vi "simple_qa_agent_sm_template.vi"   [LabVIEW 2020]
uses:
  user_interfaces/simple_html_chat_ui/simple_html_chat_ui.lvclass
  models/abstract_llm_base/abstract_llm_base.lvclass
  vectorstore/abstract_vector_base/abstract_vector_base.lvclass
  agent_simple_qa/agent_simple_qa.lvclass
  models/abstract_message_base/abstract_message_base.lvclass
  <vilib>/addons/_JKI Toolkits/State Machine/_JKI_lib_State_Machine.llb/Select State(s)_err__jki_lib_state_machine.vi
  vectorstore/vector_qdrant/vector_qdrant.lvclass
  D:/Personal/LabVIEW LLMs/src/vectorstore/abstract_vector_base/abstract_vector_base.lvclass
  models/llm_openai_chatmodels/llm_openai_chatmodels.lvclass
  D:/Personal/LabVIEW LLMs/src/models/abstract_llm_base/abstract_llm_base.lvclass
  models/llm_openai_embedding/llm_openai_embedding.lvclass
  agent_simple_qa_dynamicdata/agent_simple_qa_dynamic.lvclass
  D:/Personal/LabVIEW LLMs/src/agent/agent_simple_qa/agent_simple_qa.lvclass
  <vilib>/addons/_JKI Toolkits/State Machine/_JKI_lib_State_Machine.llb/Periodic Trigger__ogtk__JKI-SM__jki_lib_state_machine.vi
  models/llm_openai_chatmodels/Instantiate_llm_openai.vi
  models/llm_openai_embedding/Instantiate_llm_openai_embed.vi
  agent_simple_qa/poly/ask_your_model.vi
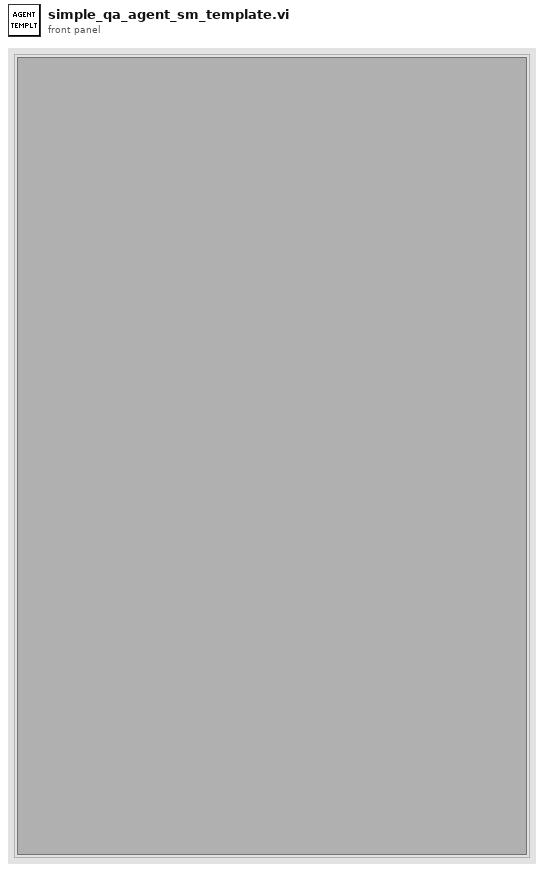
[diagram p1: front panel]
types:
  T1 = enum32{"Invalid", "Standard", "Closed", "Hidden", "Minimized", "Maximized"}
  T2 = enum32{"invalid app kind", "Development System", "Run Time System", "Student Edition", "Embedded LabVIEW", "Evaluation", "Custom"}
  T3 = cluster{"Core":cluster{"Current VI Reference":refnum<vi>, "Close Panel on Exit?":bool}, "Agent":cluster{"UI_Chat":refnum<class "simple_html_chat_ui.lvclass">, "Model_Generative":refnum<class "abstract_llm_base.lvclass">, "Model_Embedding":refnum<class "abstract_llm_base.lvclass">, "Vector Store":refnum<class "abstract_vector_base.lvclass">, "Agent_QA":refnum<class "agent_simple_qa.lvclass">, "last_message":refnum<class "abstract_message_base.lvclass">}}
  T4 = cluster{"UI_Chat":refnum<class "simple_html_chat_ui.lvclass">, "Model_Generative":refnum<class "abstract_llm_base.lvclass">, "Model_Embedding":refnum<class "abstract_llm_base.lvclass">, "Vector Store":refnum<class "abstract_vector_base.lvclass">, "Agent_QA":refnum<class "agent_simple_qa.lvclass">, "last_message":refnum<class "abstract_message_base.lvclass">}
  T5 = cluster{"Current VI Reference":refnum<vi>, "Close Panel on Exit?":bool}
  T6 = typedef "simple_html_chat_ui.lvclass/web_events.ctl" = cluster{"User prompt":refnum<user-event>, "Clear history":refnum<user-event>}
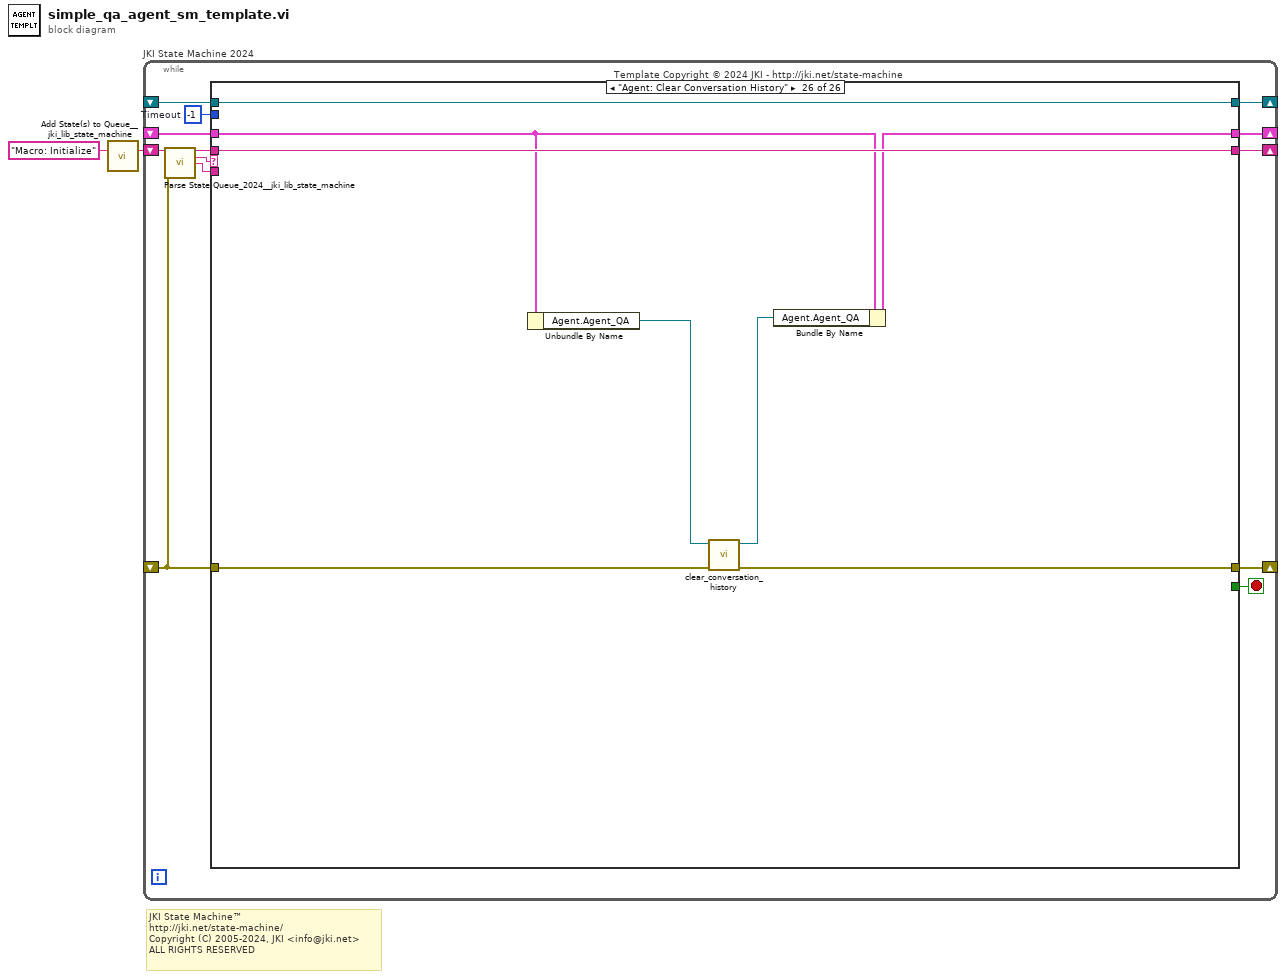
[diagram p0: block diagram]
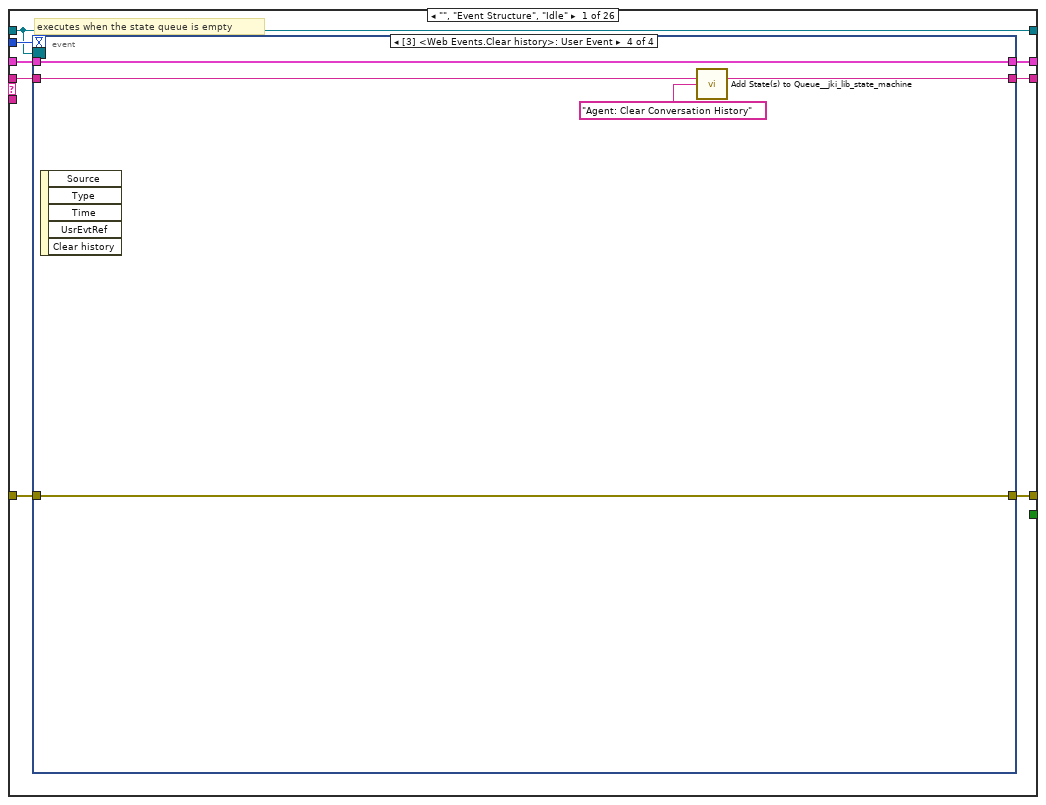
[diagram p2: hidden frame]
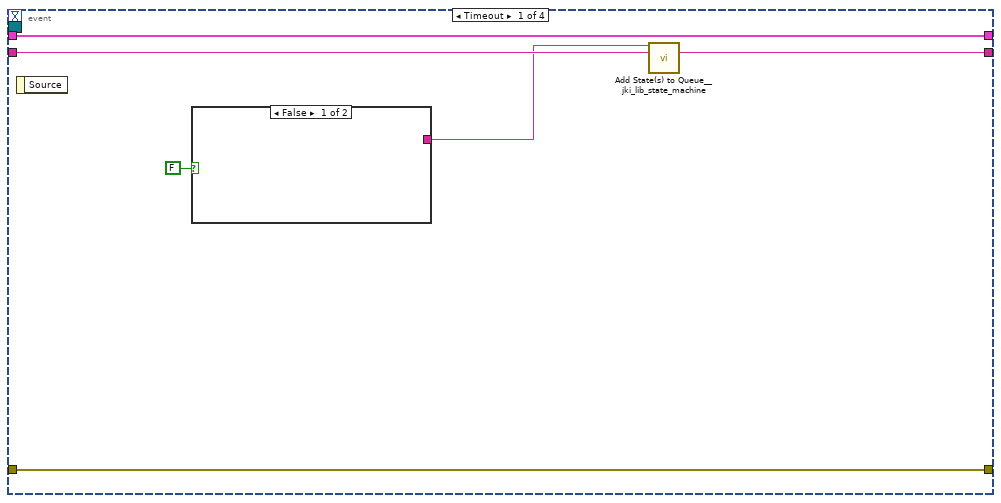
[diagram p3: hidden frame]
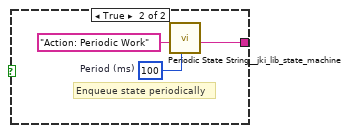
[diagram p4: hidden frame]
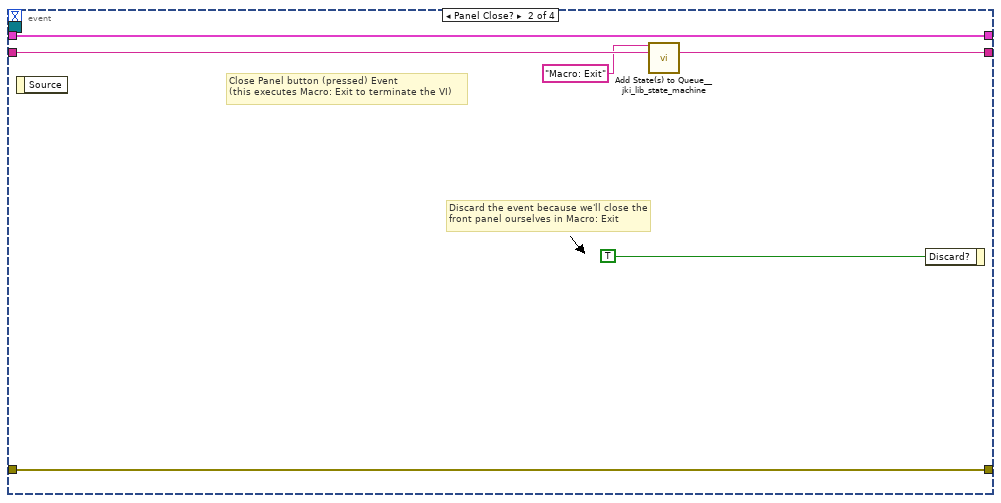
[diagram p5: hidden frame]
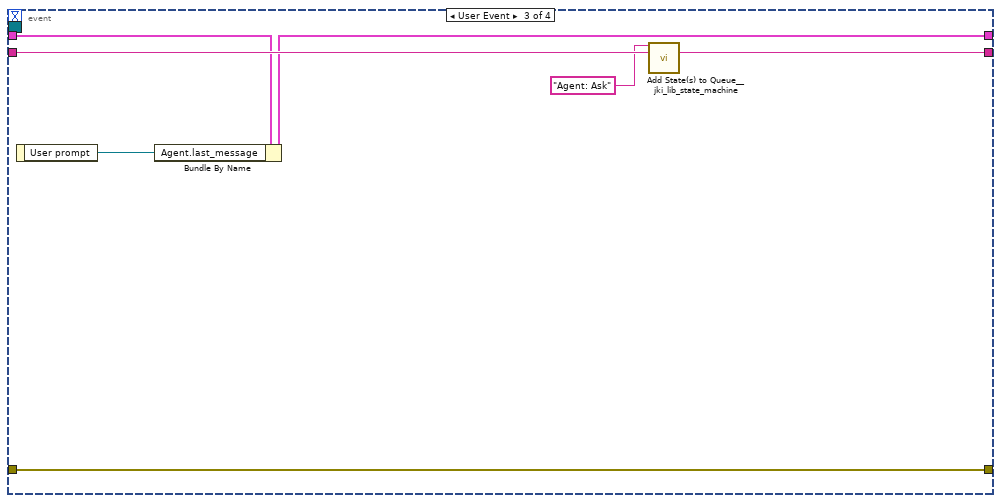
[diagram p6: hidden frame]
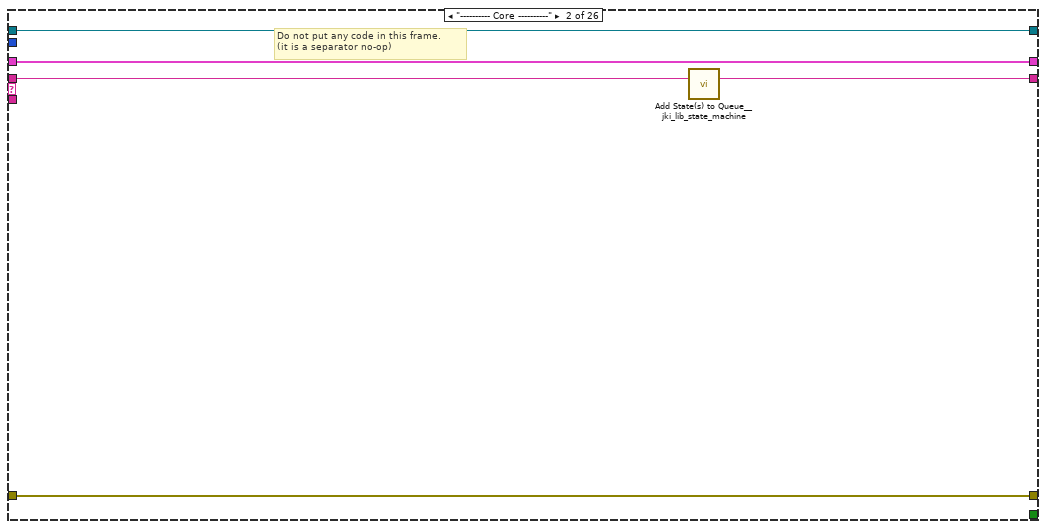
[diagram p7: hidden frame]
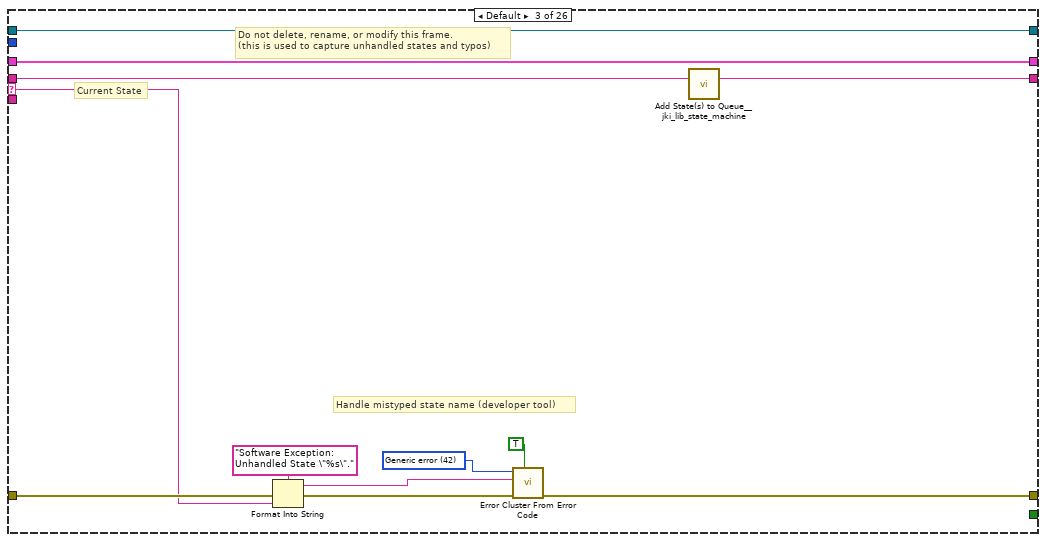
[diagram p8: hidden frame]
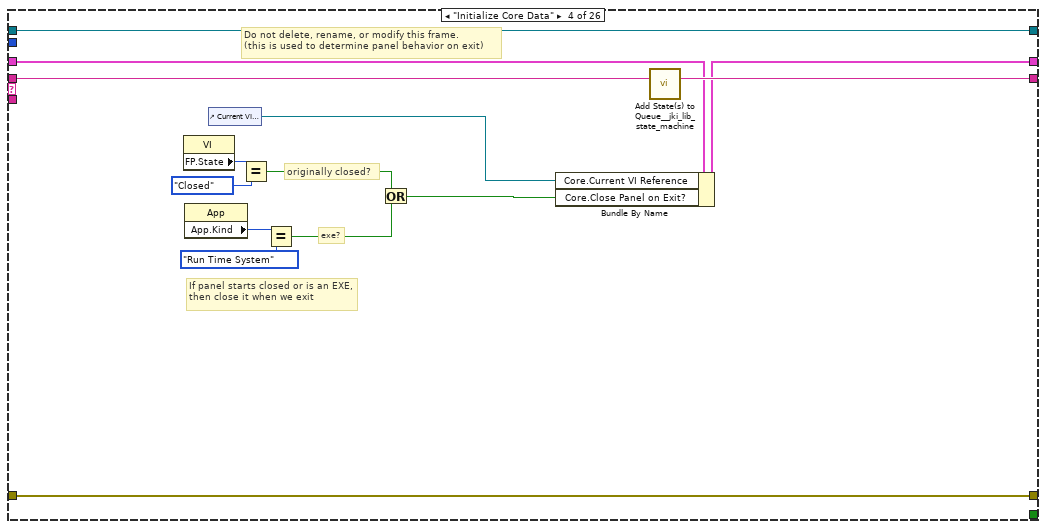
[diagram p9: hidden frame]
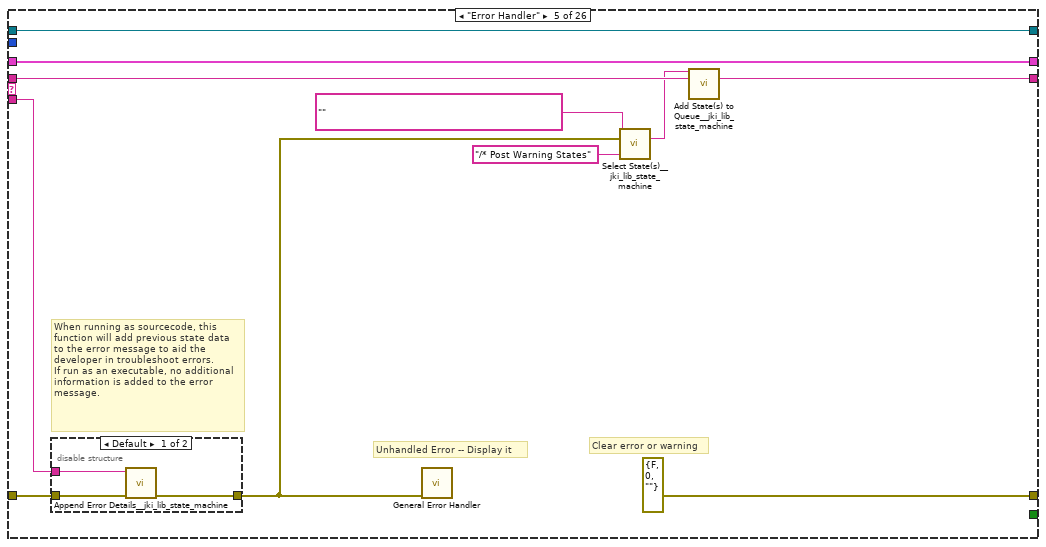
[diagram p10: hidden frame]
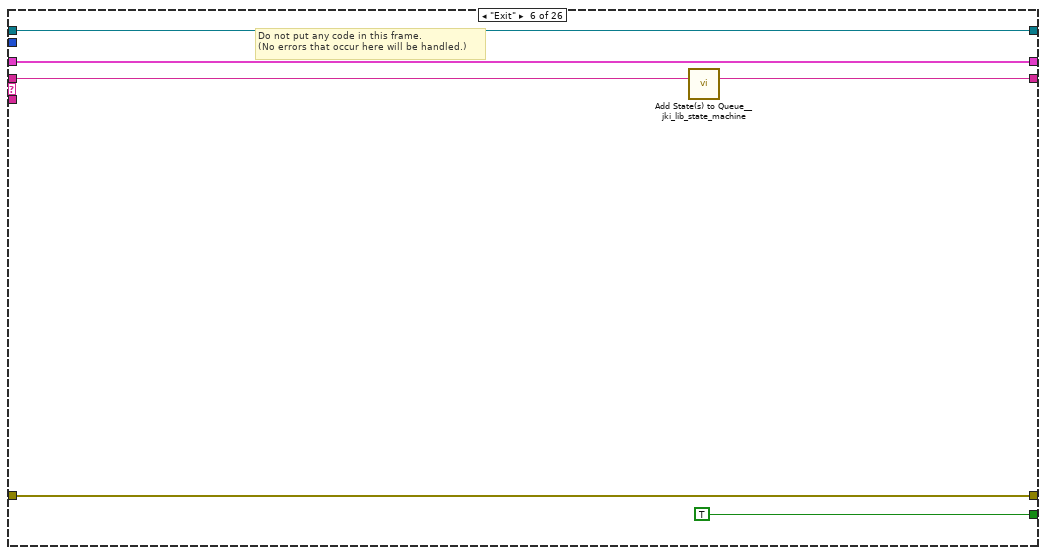
[diagram p12: hidden frame]
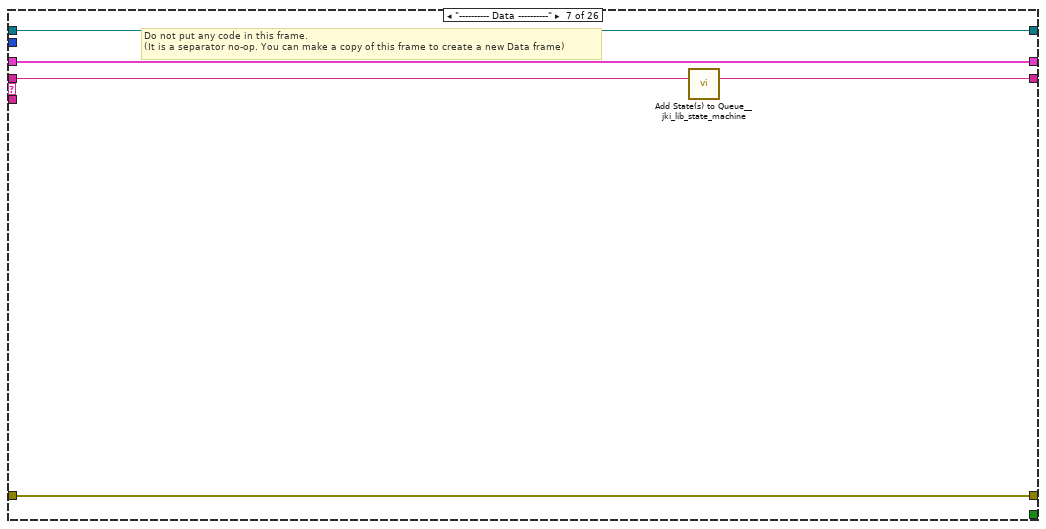
[diagram p13: hidden frame]
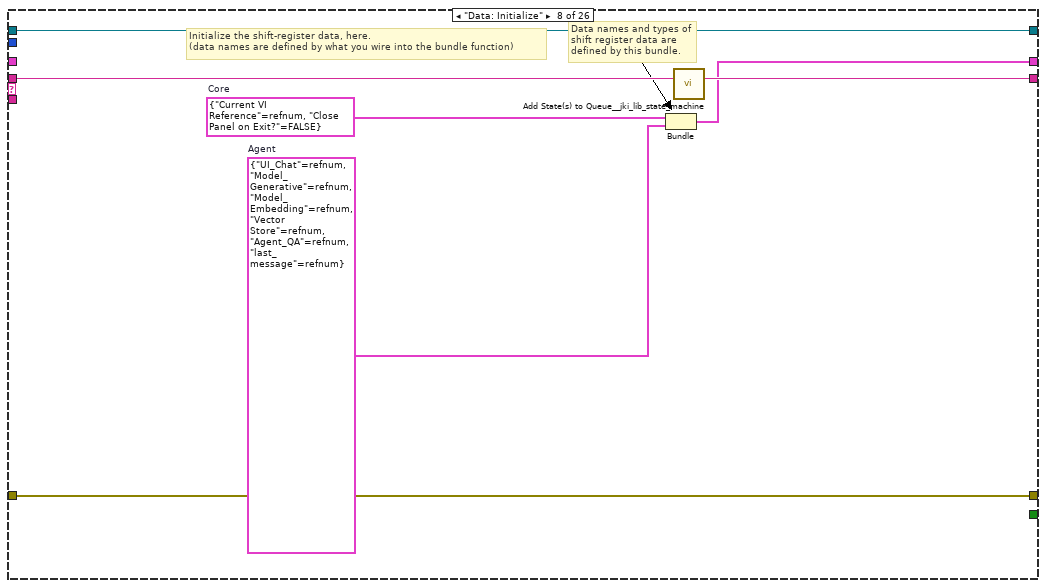
[diagram p14: hidden frame]
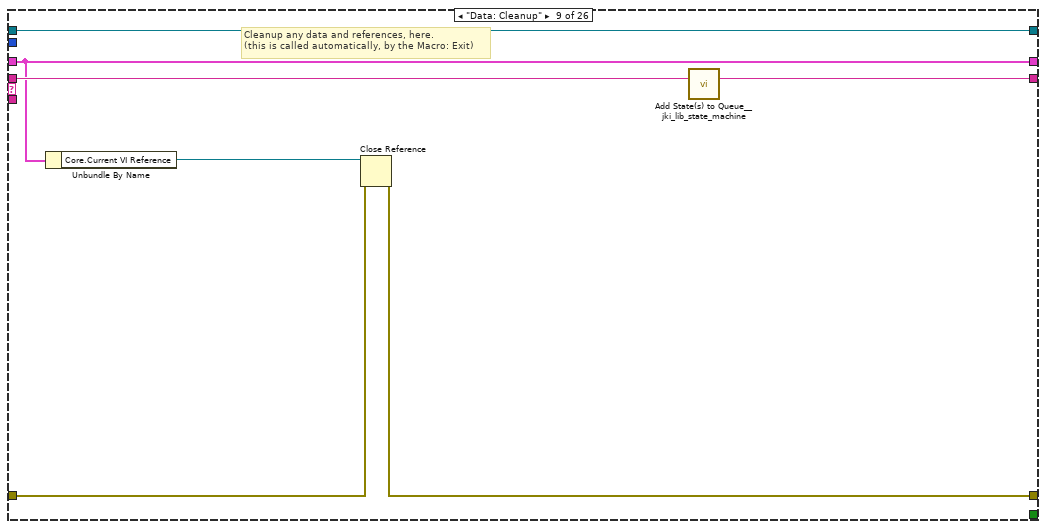
[diagram p15: hidden frame]
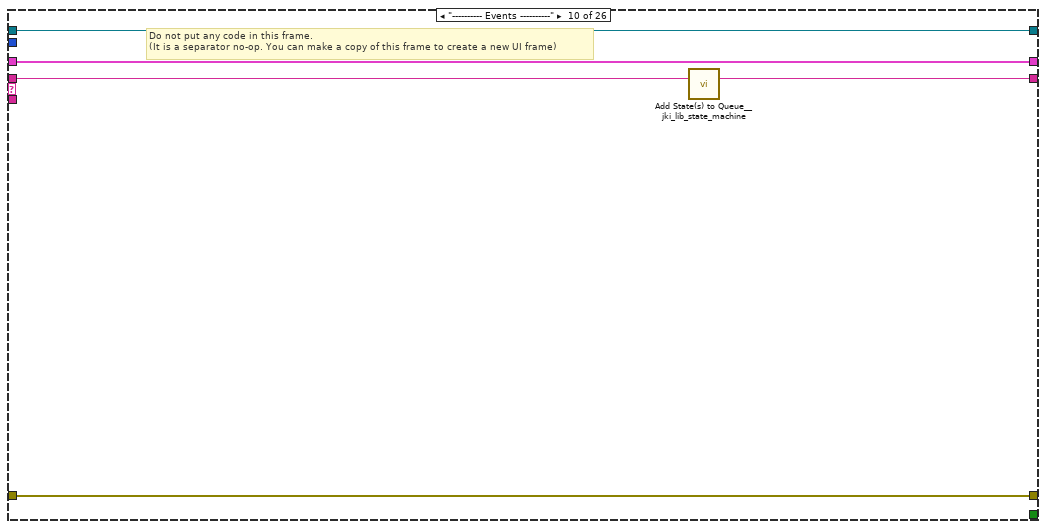
[diagram p16: hidden frame]
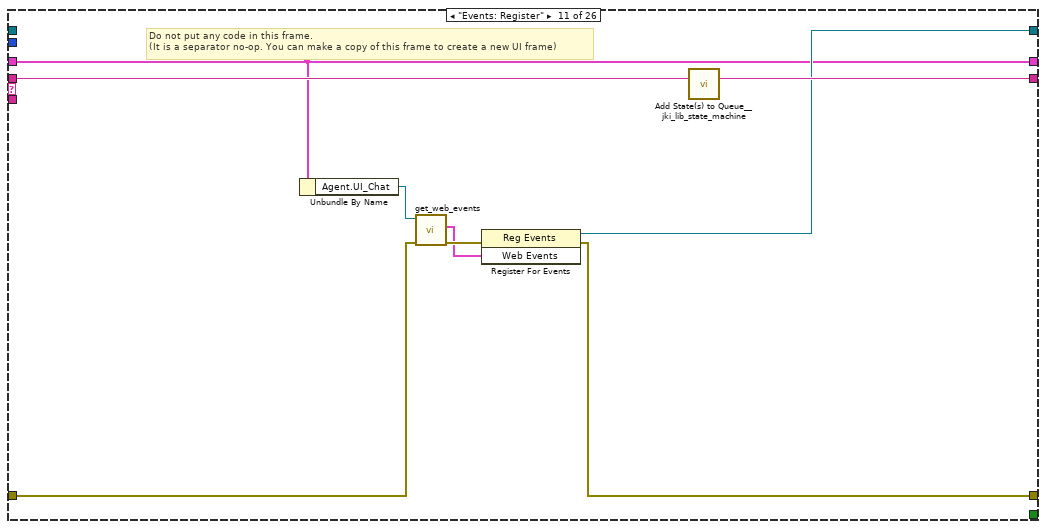
[diagram p17: hidden frame]
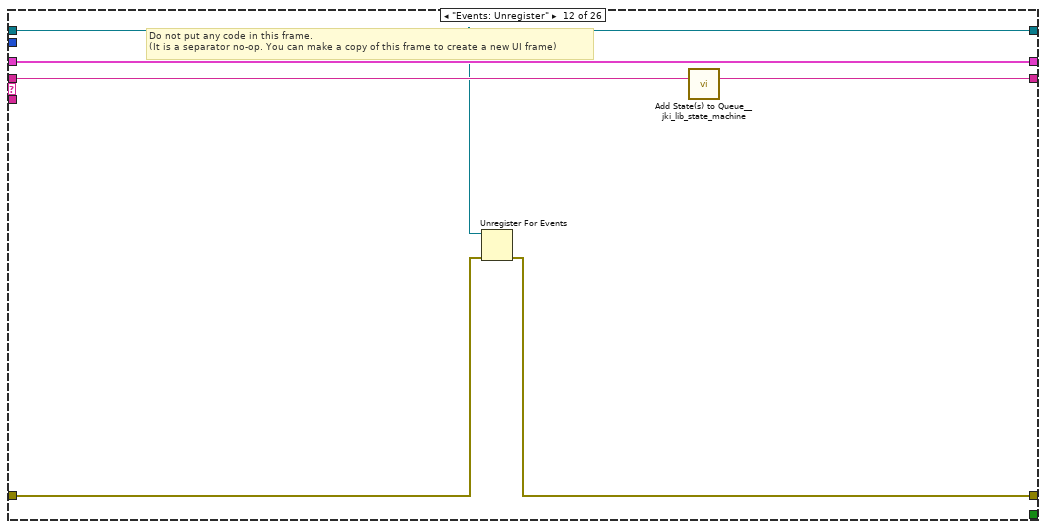
[diagram p18: hidden frame]
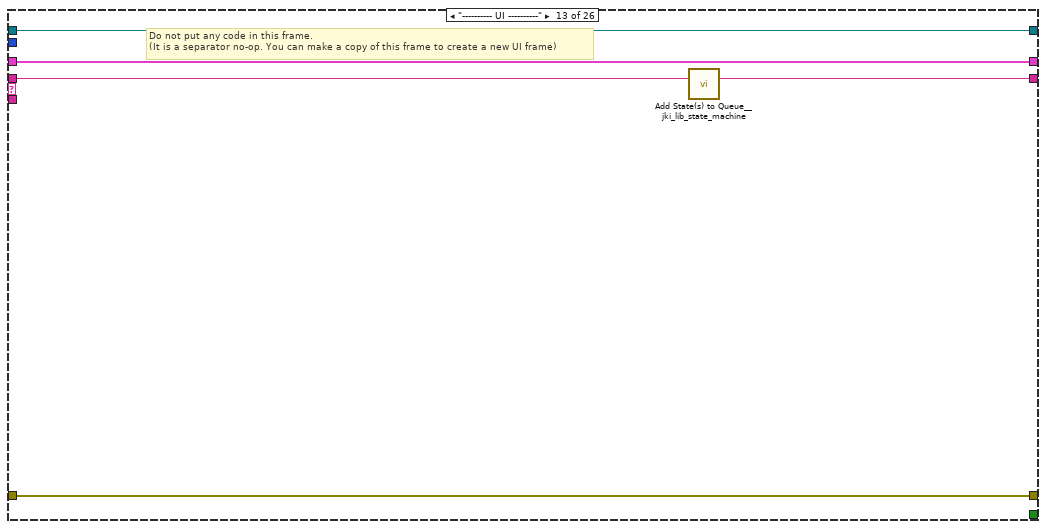
[diagram p19: hidden frame]
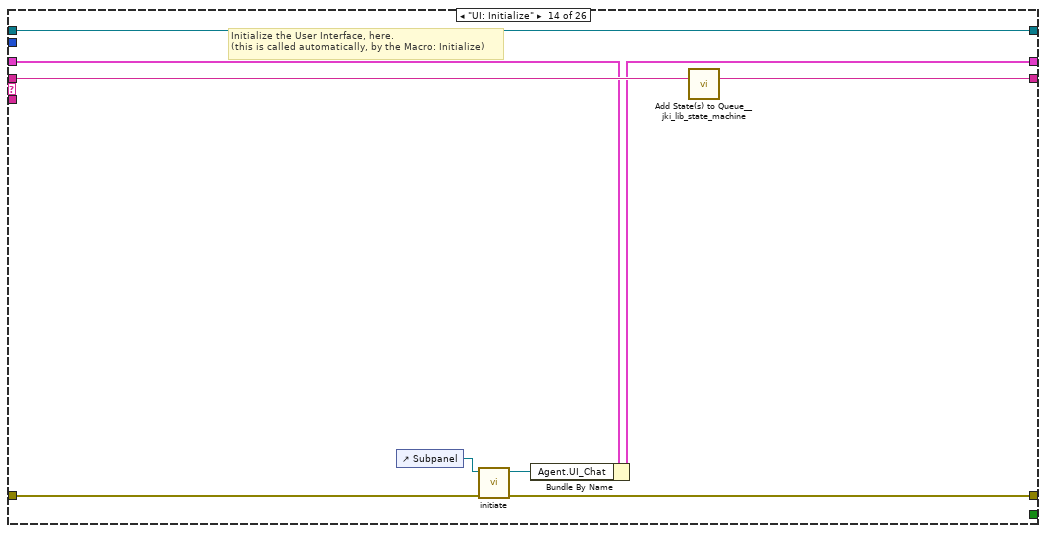
[diagram p20: hidden frame]
diagram:
  # "JKI State Machine™\nhttp://jki.net/state-machine/\nCopyright (C) 2005-2024, JKI <info@jki.net>\nALL RIGHTS RESERVED"
  n1 = call <vilib>:"Add State(s) to Queue__jki_lib_state_machine.vi"("State(s) in (\"\")"="Macro: Initialize") -> ("States Out"=w2:string)  [unwired: 14 in]
  n2 = while "JKI State Machine 2024" {
    shift-right: [w8] -> _
    shift-left: _ -> [w7]
    shift-right: [w11] -> _
    shift-left: _ -> [w5]
    shift-right: [w10] -> _
    shift-left: w2 -> [w12]
    shift-right: [w4] -> _
    shift-left: _ -> [w3]
    stop <- w9 stop-if-true
    w6 = -1  # Timeout
    # "Template Copyright © 2024 JKI - http://jki.net/state-machine"
    n3 = call <vilib>:"Parse State Queue_2024__jki_lib_state_machine.vi"("State Queue"=w12, "Error In (no error)"=w5) -> ("Remaining States"=w14:string, "Current State"=w15:string, "Arguments"=w13:string)  [unwired: 11 in]
    n4 = case shown="\"Agent: Clear Conversation History\"" w15 {
      selector: w15 -> [_ _ w57 _ _ _ _ _ _ _ _ _ _ _ _ _ _ _ _ _ _ _ _ _ _ _]
      tunnel: w14 -> [w23 w55 w61 w81 w92 w102 w107 w114 w121 w126 w135 w141 w146 w155 w162 w172 w179 w191 w261 w267 w277 w282 w307 w320 w332 w339]
      tunnel: w13 -> [_ _ _ _ w88 _ _ _ _ _ _ _ _ _ _ _ w174 w185 _ _ _ _ _ _ _ _]
      tunnel: w7 -> [w21 w52 w59 w74 w83 w100 w104 _ w116 w123 w131 w139 w143 w151 w160 w170 w177 w187 w258 w264 w275 w279 w289 w318 w327 w333]
      tunnel: [w20 w53 w63 w78 errorcluster {"status"=FALSE, "code"=0, "source"=""} ("error out") w99 w105 w111 w117 w124 w132 w136 w144 w147 w158 w166 w175 w188 w259 w265 w272 w280 w295 w312 w328 w338] -> w11
      tunnel: w5 -> [w17 w53 w62 w78 w89 w99 w105 w111 w118 w124 w130 w137 w144 w152 w159 w167 w176 w189 w259 w265 w272 w280 w293 w316 w329 w337]
      tunnel: [w22 w54 w60 w80 w91 w101 w106 w113 w120 w125 w134 w140 w145 w154 w161 w171 w178 w190 w260 w266 w276 w281 w306 w319 w331 w339] -> w10
      tunnel: [_ _ _ _ _ TRUE _ _ _ _ _ _ _ _ _ _ _ _ _ _ _ _ _ _ _ _] -> w9
      tunnel: [w19 w52 w59 w79 w83 w100 w104 w112 w116 w123 w131 w139 w143 w150 w160 w169 w177 w187 w258 w264 w275 w279 w288 w318 w325 w334] -> w8
      tunnel: w6 -> [w18 _ _ _ _ _ _ _ _ _ _ _ _ _ _ _ _ _ _ _ _ _ _ _ _ _]
      tunnel: [w16 w51 w56 w68 w82 w97 w103 w108 w115 w122 w133 w138 w142 w148 w156 w168 w173 w184 w257 w262 w268 w278 w283 w308 w321 w340] -> w4
      tunnel: w3 -> [w16 w51 w56 w68 w82 w97 w103 w108 w115 w122 _ w138 w142 w148 w156 w168 w173 w184 w257 w262 w268 w278 w283 w308 w321 w340]
      frame "", "Event Structure", "Idle" {
        # "executes when the state queue is empty"
        n5 = event shown="[3] <Web Events.Clear history>: User Event" {
          selector: w16 -> [_ _ _ _]
          dyn-events: _ -> [_ _ _ _]
          timeout: w18 -> [_ _ _ _]
          tunnel: w23 -> [w29 w38 w45 w47]
          tunnel: [w28 w37 w44 w48] -> w22
          tunnel: w21 -> [w26 w35 w42 w50]
          tunnel: [w27 w36 w40 w49] -> w20
          tunnel: w17 -> [w27 w36 w40 w49]
          tunnel: [w26 w35 w41 w50] -> w19
          event Timeout {
            n6 = event-data() -> ()  [unwired: 1 in, 1 out]
            n7 = case shown="False" FALSE {
              tunnel: [_ w32] -> w25
              frame False {
              }
              frame True {
                w30 = u32 100  # Period (ms)
                # "Enqueue state periodically"
                n8 = call <vilib>:"Periodic State String__jki_lib_state_machine.vi"("Period (ms)"=w30, "State"="Action: Periodic Work") -> ("State Out"=w32:string)  [unwired: 9 in]
              }
            }
            n9 = call <vilib>:"Add State(s) to Queue__jki_lib_state_machine.vi"("State(s) in Front (\"\")"=w25, "State(s) in (\"\")"=w29) -> ("States Out"=w28:string)  [unwired: 13 in]
          }
          event Panel Close? {
            # "Discard the event because we'll close the front panel ourselves in Macro: Exit"
            # "Close Panel button (pressed) Event\n(this executes Macro: Exit to terminate the VI)"
            n10 = event-data() -> ()  [unwired: 1 in, 1 out]
            n11 = call <vilib>:"Add State(s) to Queue__jki_lib_state_machine.vi"("State(s) in Front (\"\")"="Macro: Exit", "State(s) in (\"\")"=w38) -> ("States Out"=w37:string)  [unwired: 13 in]
            n12 = event-data("Discard?"=TRUE) -> ()  [unwired: 1 in, 1 out]
          }
          event User Event {
            n13 = event-data() -> ("User prompt"=w39:refnum<class "abstract_message_base.lvclass">)  [unwired: 1 in]
            n14 = Bundle By Name(cluster=w42, "Agent.last_message"=w39) -> (w41:T3)
            n15 = call <vilib>:"Add State(s) to Queue__jki_lib_state_machine.vi"("State(s) in Front (\"\")"="Agent: Ask", "State(s) in (\"\")"=w45) -> ("States Out"=w44:string)  [unwired: 13 in]
          }
          event User Event {
            n16 = event-data() -> ()  [unwired: 1 in, 5 out]
            n17 = call <vilib>:"Add State(s) to Queue__jki_lib_state_machine.vi"("State(s) in (\"\")"=w47, "State(s) at Back (\"\")"="Agent: Clear Conversation History" ("State(s) at Back (\"\")")) -> ("States Out"=w48:string)  [unwired: 13 in]
          }
        }
      }
      frame "---------- Core ----------" {
        # "Do not put any code in this frame.\n(it is a separator no-op)"
        n18 = call <vilib>:"Add State(s) to Queue__jki_lib_state_machine.vi"("State(s) in (\"\")"=w55) -> ("States Out"=w54:string)  [unwired: 14 in]
      }
      frame Default {
        w66 = 42 items=["No error", "Argument error", "Memory is full", "Out of zone", "End of file", "File already open", "Generic file I/O error", "File not found", "File permission error", "Disk is full", "Duplicate path", "Too many files open", "System feature not enabled", "Resource file not found", "Cannot add resource", "Resource not found", "Image not found", "Image memory error", "Pen does not exist", "Config type invalid", "Config token not found", "Config parse error", "Config memory error", "Bad external code format", "Bad external code offset", "External code not present", "Null window", "Destroy window error", "Null menu", "Print aborted", "Bad print record", "Print driver error", "Windows error during printing", "Memory error during printing", "Print dialog error", "Generic print error", "Invalid device refnum", "Device not found", "Device parameter error", "Device unit error", "Cannot open device", "Device call aborted", "Generic error", "Cancelled by user", "Object ID too low", "Object ID too high", "Object not in heap", "Unknown heap", "Unknown object (invalid DefProc)", "Unknown object (DefProc not in table)", "Message out of range", "Invalid (null) method", "Unknown message", "Manager call not supported", "Bad address", "Network operation in progress", "Network operation timed out", "Connection is busy", "Network attribute not supported", "Network error", "Address in use", "System out of memory", "Connection aborted", "Connection refused", "Not connected", "Already connected", "Connection closed", "Initialization error (interapplication manager)", "Bad occurrence", "Wait on unbound occurrence handler", "Occurrence queue overflow", "Datalog type conflict", "Unused", "Unrecognized type (interapplication manager)", "Memory corrupt", "Failed to make temporary DLL", "Old CIN version", "Drag socket not found", "Failed to load drop-object", "Failed to register OLE object", "Failed to release OLE object", "Format specifier type mismatch", "Unknown format specifier", "Too few format specifiers", "Too many format specifiers", "Scan failed", "Newer CIN version", "Error converting to variant", "Runtime menu error", "Password tampered", "Variant attribute not found", "Incompatible variant data type", "Event data is not available", "Event Store is not present", "Occurrence is not found", "Event Queue is not created", "Event info is not available", "Refnum passed is NULL", "Error retrieving Class GUID", "Error retrieving CoClass GUID", "Error retrieving TypeLib GUID.", "Bad built application magic bytes.", "Specific driver is different from the specific driver associated with the Logical Name.", "There is no session opened to the class driver.", "Max Error", "MAX - Error with config objects", "MAX - Error loading configuration", "MAX - Group not supported"]
        # "Current State"
        # "Do not delete, rename, or modify this frame.\n(this is used to capture unhandled states and typos)"
        # "Handle mistyped state name (developer tool)"
        n19 = Format Into String(format string="Software Exception: Unhandled State \"%s\"." ("message"), error in=w62, w57) -> (resulting string=w65:string, error out=w64:errorcluster)  [unwired: 1 in]
        n20 = call <vilib>:"Error Cluster From Error Code.vi"("show call chain? (False)"=TRUE, "error in (no error)"=w64, "error message (\"\")"=w65, "error code (0)"=w66) -> ("error out"=w63:errorcluster)  [unwired: 5 in]
        n21 = call <vilib>:"Add State(s) to Queue__jki_lib_state_machine.vi"("State(s) in (\"\")"=w61) -> ("States Out"=w60:string)  [unwired: 14 in]
      }
      frame "Initialize Core Data" {
        # "Do not delete, rename, or modify this frame.\n(this is used to determine panel behavior on exit)"
        # "originally closed?"
        # "exe?"
        # "If panel starts closed or is an EXE, then close it when we exit"
        n22 = property class="VI"() -> ("FP.State"=w71:T1)  [unwired: 2 in, 2 out]
        n23 = property class="App"() -> ("App.Kind"=w77:T2)  [unwired: 2 in, 2 out]
        n24 = control-ref of="Current VI Reference"() -> (w72:refnum<vi>)
        n25 = Equal?(x=w71, y=T1."Closed" ("Front Panel Window:State")) -> (x = y?=w69:bool)
        n26 = Equal?(x=w77, y=T2."Run Time System" ("Application:Kind")) -> (x = y?=w75:bool)
        n27 = Or(x=w69, y=w75) -> (x .or. y?=w73:bool)
        n28 = Bundle By Name(cluster=w74, "Core.Current VI Reference"=w72, "Core.Close Panel on Exit?"=w73) -> (w79:T3)
        n29 = call <vilib>:"Add State(s) to Queue__jki_lib_state_machine.vi"("State(s) in (\"\")"=w81) -> ("States Out"=w80:string)  [unwired: 14 in]
      }
      frame "Error Handler" {
        # "Unhandled Error -- Display it"
        # "When running as sourcecode, this function will add previous state data to the error message to aid the developer in troubleshoot errors.\nIf run as an executable, no additional information is added to the error message."
        # "Clear error or warning"
        n30 = disable-structure shown="Default" {
          disable-tunnel: w89 -> [w95 w96]
          disable-tunnel: w88 -> [w94 _]
          disable-tunnel: [w93 w96] -> w87
          frame condition #0 (active) {
            n31 = call <vilib>:"Append Error Details__jki_lib_state_machine.vi"("error in (no error)"=w95, "Previous State and Argument(s)"=w94) -> ("error out"=w93:errorcluster)  [unwired: 9 in]
          }
          frame condition #1 {
          }
        }
        n32 = call <vilib>:"General Error Handler.vi"("error in (no error)"=w87) -> ()  [unwired: 10 in, 5 out]
        n33 = call-poly <vilib>:"Select State(s)__jki_lib_state_machine.vi"("State(s) if True (\"\")"="", "Select"=w87, "State(s) if False (\"\")"="/* Post Warning States") -> ("States Out"=w85:string)  [unwired: 12 in]
        n34 = call <vilib>:"Add State(s) to Queue__jki_lib_state_machine.vi"("State(s) in Front (\"\")"=w85, "State(s) in (\"\")"=w92) -> ("States Out"=w91:string)  [unwired: 13 in]
      }
      frame "Exit" {
        # "Do not put any code in this frame.\n(No errors that occur here will be handled.)"
        n35 = call <vilib>:"Add State(s) to Queue__jki_lib_state_machine.vi"("State(s) in (\"\")"=w102) -> ("States Out"=w101:string)  [unwired: 14 in]
      }
      frame "---------- Data ----------" {
        # "Do not put any code in this frame.\n(It is a separator no-op. You can make a copy of this frame to create a new Data frame)"
        n36 = call <vilib>:"Add State(s) to Queue__jki_lib_state_machine.vi"("State(s) in (\"\")"=w107) -> ("States Out"=w106:string)  [unwired: 14 in]
      }
      frame "Data: Initialize" {
        w109 = T4 {"UI_Chat"=refnum, "Model_Generative"=refnum, "Model_Embedding"=refnum, "Vector Store"=refnum, "Agent_QA"=refnum, "last_message"=refnum}  # Agent
        w110 = T5 {"Current VI Reference"=refnum, "Close Panel on Exit?"=FALSE}  # Core
        # "Data names and types of shift register data are defined by this bundle."
        # "Initialize the shift-register data, here.\n(data names are defined by what you wire into the bundle function)"
        n37 = Bundle("Core"=w110, "Agent"=w109) -> (w112:T3)  [unwired: 1 in]
        n38 = call <vilib>:"Add State(s) to Queue__jki_lib_state_machine.vi"("State(s) in (\"\")"=w114) -> ("States Out"=w113:string)  [unwired: 14 in]
      }
      frame "Data: Cleanup" {
        # "Cleanup any data and references, here.\n(this is called automatically, by the Macro: Exit)"
        n39 = Unbundle By Name(w116) -> ("Core.Current VI Reference"=w119:refnum<vi>)
        n40 = Close Reference(reference=w119, error in (no error)=w118) -> (error out=w117:errorcluster)
        n41 = call <vilib>:"Add State(s) to Queue__jki_lib_state_machine.vi"("State(s) in (\"\")"=w121) -> ("States Out"=w120:string)  [unwired: 14 in]
      }
      frame "---------- Events ----------" {
        # "Do not put any code in this frame.\n(It is a separator no-op. You can make a copy of this frame to create a new UI frame)"
        n42 = call <vilib>:"Add State(s) to Queue__jki_lib_state_machine.vi"("State(s) in (\"\")"=w126) -> ("States Out"=w125:string)  [unwired: 14 in]
      }
      frame "Events: Register" {
        # "Do not put any code in this frame.\n(It is a separator no-op. You can make a copy of this frame to create a new UI frame)"
        n43 = Unbundle By Name(w131) -> ("Agent.UI_Chat"=w127:refnum<class "simple_html_chat_ui.lvclass">)
        n44 = call "get_web_events.vi"("error in (no error)"=w130, "simple_html_chat_ui in"=w127) -> ("error out"=w129:errorcluster, "Web Events"=w128:T6)  [unwired: 7 in, 1 out]
        n45 = register-events(error in=w129, w128) -> (reference out=w133:refnum<event-registration>, error out=w132:errorcluster)  [unwired: 1 in]
        n46 = call <vilib>:"Add State(s) to Queue__jki_lib_state_machine.vi"("State(s) in (\"\")"=w135) -> ("States Out"=w134:string)  [unwired: 14 in]
      }
      frame "Events: Unregister" {
        # "Do not put any code in this frame.\n(It is a separator no-op. You can make a copy of this frame to create a new UI frame)"
        n47 = Unregister For Events(event registration refnum=w138, error in=w137) -> (error out=w136:errorcluster)
        n48 = call <vilib>:"Add State(s) to Queue__jki_lib_state_machine.vi"("State(s) in (\"\")"=w141) -> ("States Out"=w140:string)  [unwired: 14 in]
      }
      frame "---------- UI ----------" {
        # "Do not put any code in this frame.\n(It is a separator no-op. You can make a copy of this frame to create a new UI frame)"
        n49 = call <vilib>:"Add State(s) to Queue__jki_lib_state_machine.vi"("State(s) in (\"\")"=w146) -> ("States Out"=w145:string)  [unwired: 14 in]
      }
      frame "UI: Initialize" {
        # "Initialize the User Interface, here.\n(this is called automatically, by the Macro: Initialize)"
        n50 = control-ref of="Subpanel"() -> (w149:refnum<vi>)
        n51 = call "initiate.vi"("error in"=w152, "Sub Panel"=w149) -> ("error out"=w147:errorcluster, "simple_html_chat_ui out"=w153:refnum<class "simple_html_chat_ui.lvclass">)  [unwired: 8 in]
        n52 = Bundle By Name(cluster=w151, "Agent.UI_Chat"=w153) -> (w150:T3)
        n53 = call <vilib>:"Add State(s) to Queue__jki_lib_state_machine.vi"("State(s) in (\"\")"=w155) -> ("States Out"=w154:string)  [unwired: 14 in]
      }
      frame "UI: Uninitialize" {
        # "Cleanup the User Interface, here.\n(this is called automatically, by the Macro: Exit)"
        n54 = Unbundle By Name(w160) -> ("Agent.UI_Chat"=w157:refnum<class "simple_html_chat_ui.lvclass">)
        n55 = call "destroy.vi"("error in (no error)"=w159, "simple_html_chat_ui in"=w157) -> ("error out"=w158:errorcluster)  [unwired: 8 in, 1 out]
        n56 = call <vilib>:"Add State(s) to Queue__jki_lib_state_machine.vi"("State(s) in (\"\")"=w162) -> ("States Out"=w161:string)  [unwired: 14 in]
      }
      frame "UI: UpdateAgentResponse" {
        # "Cleanup the User Interface, here.\n(this is called automatically, by the Macro: Exit)"
        n57 = Unbundle By Name(w170) -> ("Agent.last_message"=w165:refnum<class "abstract_message_base.lvclass">, "Agent.UI_Chat"=w164:refnum<class "simple_html_chat_ui.lvclass">)
        n58 = call "print_llm_response.vi"("error in (no error)"=w167, "llm_response"=w165, "simple_html_chat_ui in"=w164) -> ("error out"=w166:errorcluster, "simple_html_chat_ui out"=w163:refnum<class "simple_html_chat_ui.lvclass">)  [unwired: 7 in]
        n59 = Bundle By Name(cluster=w170, "Agent.UI_Chat"=w163) -> (w169:T3)
        n60 = call <vilib>:"Add State(s) to Queue__jki_lib_state_machine.vi"("State(s) in (\"\")"=w172) -> ("States Out"=w171:string)  [unwired: 14 in]
      }
      frame "UI: Cursor Set" {
        # "Argument"
        # "Set and Unset Cursor Busy.\n(Usage: \"UI: Cursor Set >> Busy|Idle\")"
        n61 = case shown="\"Idle\", Default" w174 {
          tunnel: w176 -> [w181 w183]
          tunnel: [w180 w182] -> w175
          frame "Idle", Default {
            n62 = call <vilib>:"Unset Busy.vi"("error in (no error)"=w181) -> ("error out"=w180:errorcluster)  [unwired: 10 in]
          }
          frame "Busy" {
            n63 = call <vilib>:"Set Busy.vi"("error in (no error)"=w183) -> ("error out"=w182:errorcluster)  [unwired: 9 in, 1 out]
          }
        }
        n64 = call <vilib>:"Add State(s) to Queue__jki_lib_state_machine.vi"("State(s) in (\"\")"=w179) -> ("States Out"=w178:string)  [unwired: 14 in]
      }
      frame "UI: Front Panel State" {
        # "Argument"
        # "Set Front Panel Open or Closed\n(Usage: \"UI: Front Panel State >> Open|Close\")"
        n65 = Unbundle By Name(w187) -> ("Core.Current VI Reference"=w186:refnum<vi>)
        n66 = case shown="\"Minimize\", \"Minimized\"" w185 {
          tunnel: w189 -> [w197 w212 w223 w236 w249]
          tunnel: [w199 w213 w225 w238 w251] -> w188
          tunnel: w186 -> [w198 w210 w224 w237 w250]
          frame "Open", "Standard", Default {
            w192 = T1."Standard" ("State")
            n67 = property class="VI"(reference=w198, error in=w197) -> (reference out=w195:refnum<vi>, error out=w196:errorcluster, "FP.State"=w194:T1)
            n68 = Not Equal?(x=w194, y=w192) -> (x != y?=w193:bool)
            n69 = case shown="True" w193 {
              tunnel: [w203 w205] -> w199
              tunnel: w196 -> [w202 w205]
              tunnel: w195 -> [w201 _]
              tunnel: w192 -> [w200 _]
              frame True {
                n70 = invoke class="VI" method="FP.Open"(reference=w201, error in=w202, "Activate"=TRUE, "State"=w200) -> (error out=w203:errorcluster)  [unwired: 1 in, 4 out]
              }
              frame False {
              }
            }
          }
          frame "Close", "Closed" {
            n71 = property class="VI"(reference=w210, error in=w212) -> (reference out=w209:refnum<vi>, error out=w211:errorcluster, "FP.State"=w207:T1)
            n72 = Not Equal?(x=w207, y=T1."Closed" ("Front Panel Window:State")) -> (x != y?=w206:bool)
            n73 = case shown="True" w206 {
              tunnel: [w214 w217] -> w213
              tunnel: w211 -> [w214 w216]
              tunnel: w209 -> [_ w215]
              frame False {
              }
              frame True {
                n74 = invoke class="VI" method="FP.Close"(reference=w215, error in=w216) -> (error out=w217:errorcluster)  [unwired: 1 in, 2 out]
              }
            }
          }
          frame "Hidden", "Hide" {
            w218 = T1."Hidden" ("State")
            n75 = property class="VI"(reference=w224, error in=w223) -> (reference out=w221:refnum<vi>, error out=w222:errorcluster, "FP.State"=w220:T1)
            n76 = Not Equal?(x=w220, y=w218) -> (x != y?=w219:bool)
            n77 = case shown="True" w219 {
              tunnel: [w229 w230] -> w225
              tunnel: w222 -> [w228 w230]
              tunnel: w221 -> [w227 _]
              tunnel: w218 -> [w226 _]
              frame True {
                n78 = invoke class="VI" method="FP.Open"(reference=w227, error in=w228, "State"=w226) -> (error out=w229:errorcluster)  [unwired: 2 in, 4 out]
              }
              frame False {
              }
            }
          }
          frame "Minimize", "Minimized" {
            w231 = T1."Minimized" ("State")
            n79 = property class="VI"(reference=w237, error in=w236) -> (reference out=w234:refnum<vi>, error out=w235:errorcluster, "FP.State"=w233:T1)
            n80 = Not Equal?(x=w233, y=w231) -> (x != y?=w232:bool)
            n81 = case shown="True" w232 {
              tunnel: [w242 w243] -> w238
              tunnel: w235 -> [w241 w243]
              tunnel: w234 -> [w240 _]
              tunnel: w231 -> [w239 _]
              frame True {
                n82 = invoke class="VI" method="FP.Open"(reference=w240, error in=w241, "State"=w239) -> (error out=w242:errorcluster)  [unwired: 2 in, 4 out]
              }
              frame False {
              }
            }
          }
          frame "Maximize", "Maximized" {
            w244 = T1."Maximized" ("State")
            n83 = property class="VI"(reference=w250, error in=w249) -> (reference out=w247:refnum<vi>, error out=w248:errorcluster, "FP.State"=w246:T1)
            n84 = Not Equal?(x=w246, y=w244) -> (x != y?=w245:bool)
            n85 = case shown="True" w245 {
              tunnel: [w255 w256] -> w251
              tunnel: w248 -> [w254 w256]
              tunnel: w247 -> [w253 _]
              tunnel: w244 -> [w252 _]
              frame True {
                n86 = invoke class="VI" method="FP.Open"(reference=w253, error in=w254, "State"=w252) -> (error out=w255:errorcluster)  [unwired: 2 in, 4 out]
              }
              frame False {
              }
            }
          }
        }
        n87 = call <vilib>:"Add State(s) to Queue__jki_lib_state_machine.vi"("State(s) in (\"\")"=w191) -> ("States Out"=w190:string)  [unwired: 14 in]
      }
      frame "---------- Macro ----------" {
        # "Do not put any code in this frame.\n(It is a separator no-op. You can make a copy of this frame to create a new Macro frame)"
        n88 = call <vilib>:"Add State(s) to Queue__jki_lib_state_machine.vi"("State(s) in (\"\")"=w261) -> ("States Out"=w260:string)  [unwired: 14 in]
      }
      frame "Macro: Initialize" {
        # "Initialization Macro\n(This is called once, when the VI starts)"
        n89 = call <vilib>:"Add State(s) to Queue__jki_lib_state_machine.vi"("State(s) in Front (\"\")"="Data: Initialize\nInitialize Core Data\nUI: Initialize\nEvents: Register\nUI: Front Panel State >> Open\n\nAgent: Initialize", "State(s) in (\"\")"=w267) -> ("States Out"=w266:string)  [unwired: 13 in]
      }
      frame "Macro: Exit" {
        # "Exit Macro\n(This is called once, when the VI exits)"
        n90 = Unbundle By Name(w275) -> ("Core.Close Panel on Exit?"=w270:bool)
        n91 = call <vilib>:"Conditional State String__jki_lib_state_machine.vi"("Do State(s)?"=w270, "State"="UI: Front Panel State >> Close") -> ("State Out"=w269:string)  [unwired: 7 in]
        n92 = call <vilib>:"Add State(s) to Queue__jki_lib_state_machine.vi"("State(s) in (\"\")"=w269, "State(s) at Back (\"\")"="UI: Uninitialize\nData: Cleanup\nEvents: Unregister\n\nAgent: Close\n\nExit") -> ("States Out"=w273:string)  [unwired: 13 in]
        n93 = call <vilib>:"Add State(s) to Queue__jki_lib_state_machine.vi"("State(s) in Front (\"\")"=w273, "State(s) in (\"\")"=w277) -> ("States Out"=w276:string)  [unwired: 13 in]
      }
      frame "----------Agents----------" {
        # "Template Separator\n(You can make a copy of, or modify, this frame)"
        n94 = call <vilib>:"Add State(s) to Queue__jki_lib_state_machine.vi"("State(s) in (\"\")"=w282) -> ("States Out"=w281:string)  [unwired: 14 in]
      }
      frame "Agent: Initialize" {
        w296 = FALSE  # skip_loading_data
        # "Your code here.\n(You can make a copy of, or modify, this frame)"
        n95 = call "get_env_variable.vi"("Environment Variable Name"="labview_llm_openai_key") -> ("Value"=w303:string)  [unwired: 1 in, 1 out]
        n96 = call "get_env_variable.vi"("Environment Variable Name"="labview_llm_openai_key") -> ("Value"=w298:string)  [unwired: 1 in, 1 out]
        n97 = call "instantiate_qdrant_vector.vi"("host_url"="http://10.0.0.209:6333/", "error in"=w293) -> ("vector_qdrant out"=w286:refnum<class "vector_qdrant.lvclass">, "error out"=w291:errorcluster)  [unwired: 12 in]
        n98 = call-poly "instantiate_chat_model.vi"("model_name"="gpt-4o-mini", "openai_key"=w303, "error in (no error)"=w293) -> ("llm_openai out"=w285:refnum<class "llm_openai_chatmodels.lvclass">, "error out"=w290:errorcluster)  [unwired: 11 in]
        n99 = call-poly "instantiate_embedding_model.vi"("model_name"="text-embedding-ada-002", "openai_key"=w298, "error in (no error)"=w293) -> ("llm_openai_embedding out"=w284:refnum<class "llm_openai_embedding.lvclass">, "error out"=w294:errorcluster)  [unwired: 11 in]
        n100 = Merge Errors(w291, w290, w294) -> (w292:errorcluster)
        n101 = call "instantiate_simple_qa_dynamic.vi"("vectorestore"=w286, "skip_loading_data"=w296, "collection_name"="example_pipeline_collection" ("host_url"), "chat_model"=w285, "embedding_model"=w284, "error in (no error)"=w292, "sources"=string[] [] ("webpages")) -> ("agent_webpage_qa out"=w287:refnum<class "agent_simple_qa_dynamic.lvclass">, "error out"=w295:errorcluster)  [unwired: 7 in]
        n102 = call <vilib>:"Add State(s) to Queue__jki_lib_state_machine.vi"("State(s) in (\"\")"=w307) -> ("States Out"=w306:string)  [unwired: 14 in]
        n103 = Bundle By Name(cluster=w289, "Agent.Vector Store"=w286, "Agent.Model_Generative"=w285, "Agent.Model_Embedding"=w284, "Agent.Agent_QA"=w287) -> (w288:T3)
      }
      frame "Agent: Close" {
        # "Your code here.\n(You can make a copy of, or modify, this frame)"
        n104 = Unbundle By Name(w318) -> ("Agent.Model_Generative"=w309:refnum<class "abstract_llm_base.lvclass">, "Agent.Model_Embedding"=w310:refnum<class "abstract_llm_base.lvclass">, "Agent.Vector Store"=w311:refnum<class "abstract_vector_base.lvclass">, "Agent.Agent_QA"=w317:refnum<class "agent_simple_qa.lvclass">)
        n105 = call-dynamic "destroy.vi"("agent_simple_qa in"=w317, "error in (no error)"=w316) -> ("error out"=w315:errorcluster)  [unwired: 12 in, 1 out]
        n106 = call-dynamic "destroy.vi"("abstract_vector_base in"=w311, "error in (no error)"=w315) -> ("error out"=w314:errorcluster)  [unwired: 12 in, 1 out]
        n107 = call-dynamic "destroy.vi"("error in (no error)"=w314, "abstract_llm_base in"=w310) -> ("error out"=w313:errorcluster)  [unwired: 8 in, 1 out]
        n108 = call-dynamic "destroy.vi"("error in (no error)"=w313, "abstract_llm_base in"=w309) -> ("error out"=w312:errorcluster)  [unwired: 8 in, 1 out]
        n109 = call <vilib>:"Add State(s) to Queue__jki_lib_state_machine.vi"("State(s) in (\"\")"=w320) -> ("States Out"=w319:string)  [unwired: 14 in]
      }
      frame "Agent: Ask" {
        n110 = Unbundle By Name(w327) -> ("Agent.last_message"=w324:refnum<class "abstract_message_base.lvclass">, "Agent.Agent_QA"=w330:refnum<class "agent_simple_qa.lvclass">)
        n111 = call-poly "ask_poly.vi"("error in (no error)"=w329, "message"=w324, "agent_simple_qa in"=w330) -> ("error out"=w328:errorcluster, "message_response"=w323:refnum<class "abstract_message_base.lvclass">, "agent_simple_qa out"=w326:refnum<class "agent_simple_qa.lvclass">)  [unwired: 6 in]
        n112 = Bundle By Name(cluster=w327, "Agent.last_message"=w323, "Agent.Agent_QA"=w326) -> (w325:T3)
        n113 = call <vilib>:"Add State(s) to Queue__jki_lib_state_machine.vi"("State(s) in Front (\"\")"="UI: UpdateAgentResponse" ("State(s) in Front (\"\")"), "State(s) in (\"\")"=w332) -> ("States Out"=w331:string)  [unwired: 13 in]
      }
      frame "Agent: Clear Conversation History" {
        n114 = Unbundle By Name(w333) -> ("Agent.Agent_QA"=w336:refnum<class "agent_simple_qa.lvclass">)
        n115 = call-dynamic "clear_conversation_history.vi"("error in (no error)"=w337, "agent_simple_qa in"=w336) -> ("error out"=w338:errorcluster, "agent_simple_qa out"=w335:refnum<class "agent_simple_qa.lvclass">)  [unwired: 8 in]
        n116 = Bundle By Name(cluster=w333, "Agent.Agent_QA"=w335) -> (w334:T3)
      }
    }
  }
